vi "serial_arduino.vi"() -> ()   [LabVIEW 2016]
uses:
  <vilib>/Instr/_visa.llb/VISA Configure Serial Port (Instr).vi
panel:
  in  "stop":bool
  in  "Send":bool
  in  "VISA resource name":refnum<visa-resource-name>
  out "Response":string
  in  "Sent":string
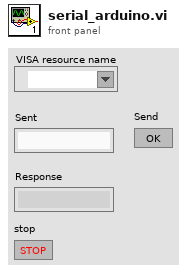
[diagram p1: front panel]
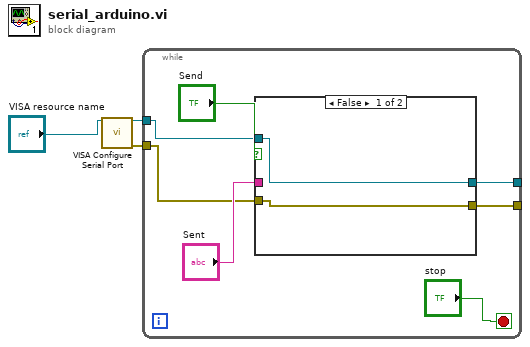
[diagram p0: block diagram]
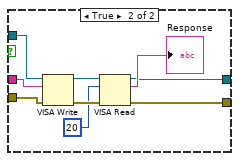
[diagram p2: hidden frame]
diagram:
  n1 = call-poly "VISA Configure Serial Port"("VISA resource name"="VISA resource name") -> ("VISA resource name out"=w1:refnum<visa-resource-name>, "error out"=w2:errorcluster)  [unwired: 13 in]
  n2 = while {
    tunnel: [w7] -> _
    tunnel: [w6] -> _
    tunnel: w2 -> [w5]
    tunnel: w1 -> [w4]
    stop <- "stop" stop-if-true
    n3 = case shown="False" "Send" {
      tunnel: "Sent" -> [_ w21]
      tunnel: [w11 w17] -> w7
      tunnel: [w12 w16] -> w6
      tunnel: w5 -> [w12 w14]
      tunnel: w4 -> [w11 w13]
      frame False {
      }
      frame True {
        n4 = VISA Write(VISA resource name=w13, write buffer=w21, error in (no error)=w14) -> (VISA resource name out=w19:refnum<visa-resource-name>, error out=w20:errorcluster)  [unwired: 1 out]
        n5 = VISA Read(VISA resource name=w19, byte count=20, error in (no error)=w20) -> (VISA resource name out=w17:refnum<visa-resource-name>, read buffer=→"Response":string, error out=w16:errorcluster)  [unwired: 1 out]
      }
    }
  }
